vi "Check.vi"(8 "Error In":errorcluster, 11 "reference in":refnum<class "Heartbeat.lvclass">) -> (0 "Error Out":errorcluster, 1 "Emergency?":bool[](array[boolean]), 2 "Nodes":u8[](array[numeric]), 3 "reference out":refnum<class "Heartbeat.lvclass">)   [LabVIEW 2024, in "CANopen Master.lvlib" / "Heartbeat.lvclass"]
uses:
  Heartbeat.lvclass
  Heartbeat.lvclass/Heartbeat.ctl
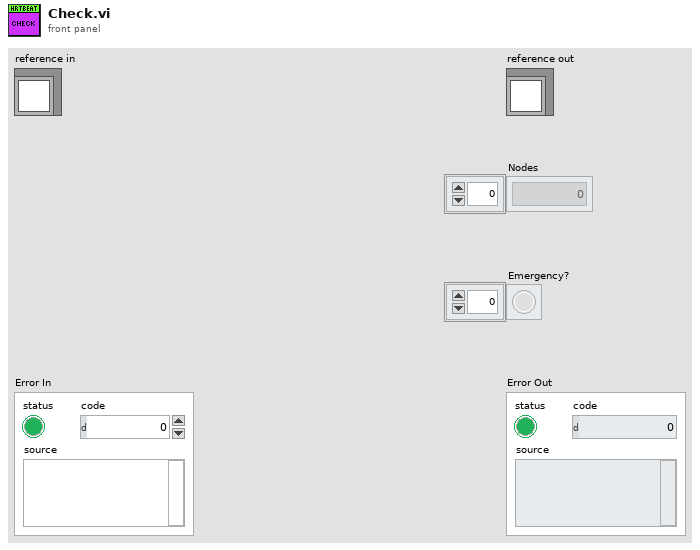
[diagram p1: front panel]
types:
  T1 = typedef "CANopen Master.lvlib/Heartbeat.lvclass/ObjectAttributes.ctl" = cluster{"Heartbeats":map{u8, cluster{"Period":u16, "Timeout":u16, "Last Beat":timestamp}}}
  T2 = map{u8, cluster{"Period":u16, "Timeout":u16, "Last Beat":timestamp}}
  T3 = cluster{"Period":u16, "Timeout":u16, "Last Beat":timestamp}
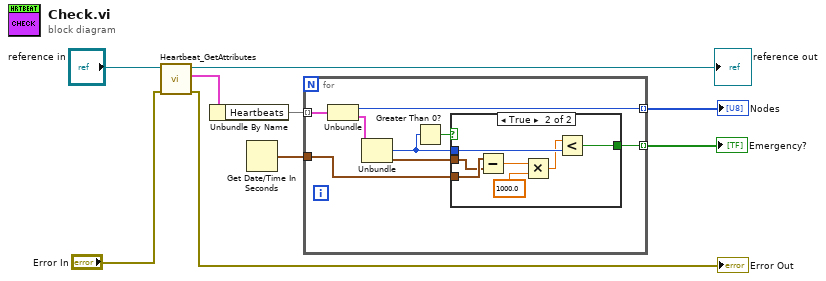
[diagram p0: block diagram]
diagram:
  n1 = call "Heartbeat_GetAttributes.vi"("Error In"="Error In", "reference in"="reference in") -> ("Error Out"=→"Error Out":errorcluster, "Data"=w5:T1, "reference out"=→"reference out":refnum<class "Heartbeat.lvclass">)  [unwired: 6 in, 1 out]
  n2 = Unbundle By Name(w5) -> ("Heartbeats"=w4:T2)
  n3 = Get Date/Time In Seconds() -> (seconds since 1Jan1904=w2:timestamp)
  n4 = for {
    tunnel: w4 -> [w17] mode=indexing
    tunnel: [w14] -> w6 mode=indexing
    tunnel: [w13] -> w7 mode=indexing
    tunnel: w2 -> [w12]
    n5 = Unbundle(w17) -> ("Node-ID"=w13:u8, "Value"=w16:T3)
    n6 = Unbundle(w16) -> ("Timeout"=w11:u16, "Last Beat"=w15:timestamp)  [unwired: 1 out]
    n7 = Greater Than 0?(x=w11) -> (x > 0?=w10:bool)
    n8 = case shown="True" w10 {
      tunnel: w15 -> [_ w21]
      tunnel: w11 -> [_ w24]
      tunnel: [_ w23] -> w14
      tunnel: w12 -> [_ w22]
      frame False {
      }
      frame True {
        n9 = Subtract(x=w22, y=w21) -> (x-y=w20:dbl)
        n10 = Multiply(x=w20, y=1000.0) -> (x*y=w19:dbl)
        n11 = Less?(x=w19, y=w24) -> (x < y?=w23:bool)
      }
    }
  }
  "Nodes" <- w7
  "Emergency?" <- w6
